vi "Update Attributes Transport and VI Ref.vi"(7 "Attributes in":refnum<class "Attributes.lvclass">, 9 "VI Ref":refnum<vi>, 10 "Transport":refnum<class "Transport.lvclass">) -> (0 "Error out":errorcluster, 5 "Attributes out":refnum<class "Attributes.lvclass">)   [LabVIEW 2020, in "jettl.lvlib"]
uses:
  jettl.lvlib
  Attributes/Attributes.lvclass
  Transport/Transport.lvclass
  Attributes.ctl
  Attributes Metadata/Attributes Metadata.lvclass
  Msgs.ctl
  Msg/Msg.lvclass
  Actor/Actor.lvclass
  Base Attributes/Base Attributes.lvlib
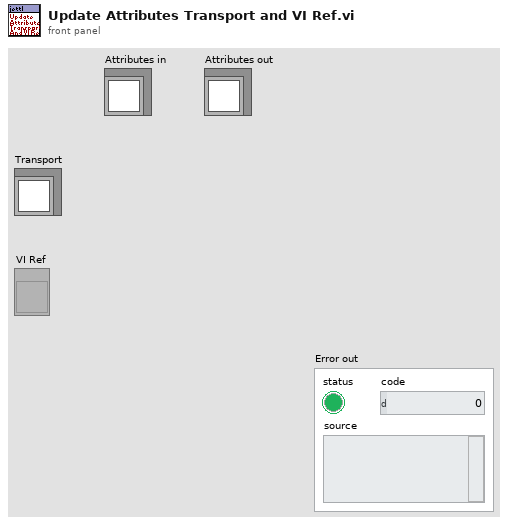
[diagram p1: front panel]
types:
  T1 = typedef "jettl.lvlib/Attributes.ctl" = cluster{"Attributes Metadata":refnum<class "Attributes Metadata.lvclass">, "Unified Msgs":T2, "Unified Leaf":bool, "Edge Actors":refnum<class "Actor.lvclass">[], "Core Actors":refnum<class "Actor.lvclass">[], "Parent Attributes":refnum<class "Attributes.lvclass">, "Root":bool, "UID":string, "Transport":refnum<class "Transport.lvclass">, "VI Ref":refnum<vi>, "Actors":refnum<class "Actor.lvclass">[]}
  T2 = typedef "jettl.lvlib/Msgs.ctl" = set{refnum<class "Msg.lvclass">}
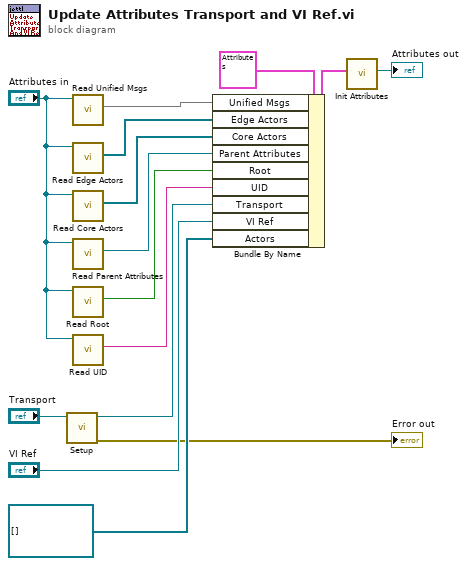
[diagram p0: block diagram]
diagram:
  n1 = call-dynamic "Setup.vi"("Transport in"="Transport") -> ("Error out"=→"Error out":errorcluster, "Transport out"=w1:refnum<class "Transport.lvclass">)  [unwired: 9 in]
  n2 = call-dynamic "Read Unified Msgs.vi"("Attributes in"="Attributes in") -> ("Unified Msgs"=w5:T2)  [unwired: 10 in]
  n3 = call-dynamic "Read Edge Actors.vi"("Attributes in"="Attributes in") -> ("Edge Actors"=w4:refnum<class "Actor.lvclass">[])  [unwired: 10 in]
  n4 = call-dynamic "Read Core Actors.vi"("Attributes in"="Attributes in") -> ("Core Actors"=w9:refnum<class "Actor.lvclass">[])  [unwired: 10 in]
  n5 = call-dynamic "Read Parent Attributes.vi"("Attributes in"="Attributes in") -> ("Parent Attributes"=w10:refnum<class "Attributes.lvclass">)  [unwired: 10 in]
  n6 = call-dynamic "Read Root.vi"("Attributes in"="Attributes in") -> ("Root"=w11:bool)  [unwired: 10 in]
  n7 = call-dynamic "Read UID.vi"("Attributes in"="Attributes in") -> ("UID"=w12:string)  [unwired: 10 in]
  n8 = Bundle By Name(cluster=T1 {"Attributes Metadata"=refnum, "Unified Msgs"={}, "Unified Leaf"=FALSE, "Edge Actors"=[], "Core Actors"=[], "Parent Attributes"=refnum, "Root"=FALSE, "UID"="", "Transport"=refnum, "VI Ref"=refnum, "Actors"=[]} ("Attributes"), "Unified Msgs"=w5, "Edge Actors"=w4, "Core Actors"=w9, "Parent Attributes"=w10, "Root"=w11, "UID"=w12, "Transport"=w1, "VI Ref"="VI Ref", "Actors"=refnum<class "Actor.lvclass">[] []) -> (w13:T1)
  n9 = call "Init Attributes.vi"("Attributes"=w13) -> ("Attributes"=→"Attributes out":refnum<class "Attributes.lvclass">)  [unwired: 10 in]
